vi "cg_Bracket Fletcher.vi"(4 "p":dbl[](array[numeric]) format="%.2f", 6 "loops":u32, 7 "function and data":T1, 8 "error in (no error)":errorcluster, 9 "xit":dbl[](array[numeric]) format="%.2f", 10 "b (start)":dbl format="%.2f", 11 "a (start)":dbl format="%.2f") -> (0 "error out":errorcluster, 1 "c (bracket)":dbl format="%.2f", 2 "b (bracket)":dbl format="%.2f", 3 "a (bracket)":dbl format="%.2f", 5 "number of function calls":i32)   [LabVIEW 2017, in "NI_Gmath.lvlib"]
uses:
  NI_Gmath.lvlib
  ucno_user function ref and data.ctl
  ucno_user objective function ref.ctl
panel:
  out "error":i32
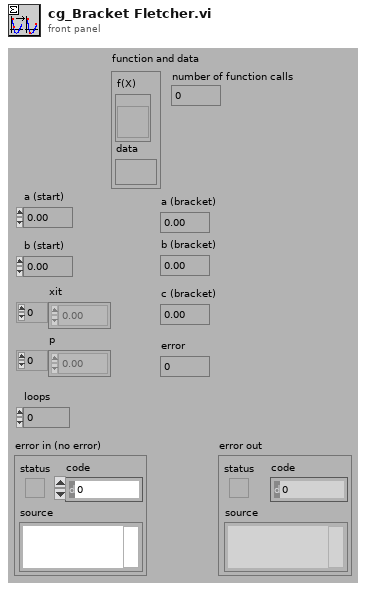
[diagram p1: front panel]
types:
  T1 = typedef "NI_Gmath.lvlib/ucno_user function ref and data.ctl" = cluster{"f(X)":T2, "data":variant}
  T2 = typedef "NI_Gmath.lvlib/ucno_user objective function ref.ctl" = refnum<vi>
  T3 = cluster{"objective function":bool, "gradient":bool}
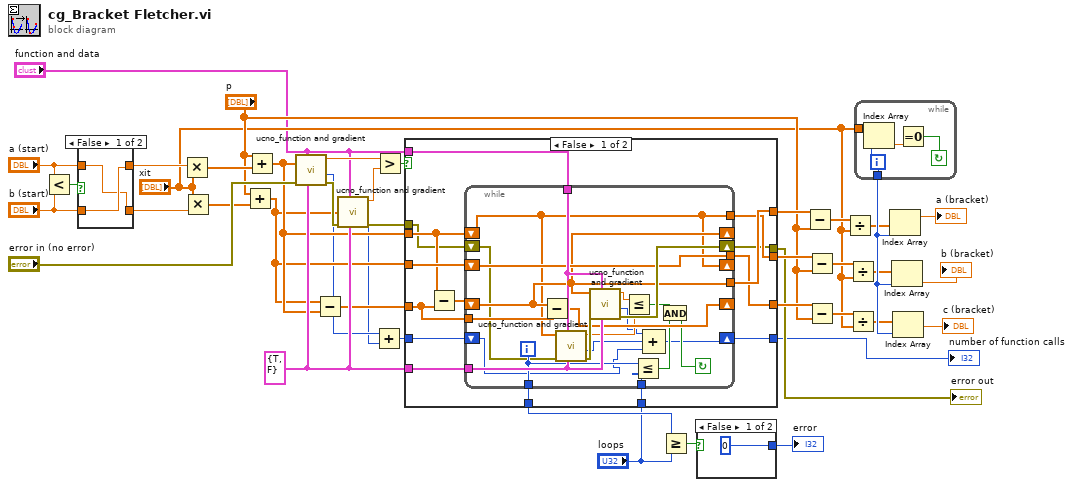
[diagram p0: block diagram]
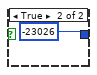
[diagram p3: hidden frame]
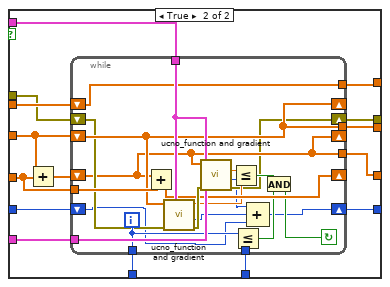
[diagram p4: hidden frame]
diagram:
  w42 = T3 {"objective function"=TRUE, "gradient"=FALSE} ("output control")
  n1 = Less?(x="a (start)", y="b (start)") -> (x < y?=w33:bool)
  n2 = case shown="False" w33 {
    tunnel: "a (start)" -> [w43 w46]
    tunnel: [w44 w46] -> w29
    tunnel: "b (start)" -> [w44 w45]
    tunnel: [w43 w45] -> w26
    frame False {
    }
    frame True {
    }
  }
  n3 = Multiply(x=w29, y="xit") -> (x*y=w28:dbl[])
  n4 = Multiply(x="xit", y=w26) -> (x*y=w25:dbl[])
  n5 = Add(x="p", y=w25) -> (x+y=w24:dbl[])
  n6 = Add(x="p", y=w28) -> (x+y=w27:dbl[])
  n7 = call "ucno_function and gradient.vi"("output control"=w42, "function and data"="function and data", "error in (no error)"="error in (no error)", "X"=w27) -> ("error out"=w41:errorcluster, "number of function calls"=w4:i32, "f(X)"=w8:dbl)  [unwired: 4 in, 1 out]
  n8 = Subtract(x=w24, y=w27) -> (x-y=w38:dbl[])
  n9 = call "ucno_function and gradient.vi"("output control"=w42, "function and data"="function and data", "error in (no error)"=w41, "X"=w24) -> ("error out"=w7:errorcluster, "number of function calls"=w3:i32, "f(X)"=w31:dbl)  [unwired: 4 in, 1 out]
  n10 = Add(x=w4, y=w3) -> (x+y=w2:i32)
  n11 = Greater?(x=w8, y=w31) -> (0:w39:bool)
  n12 = case shown="False" w39 {
    tunnel: w27 -> [w58 w97]
    tunnel: w24 -> [w59 w96]
    tunnel: w38 -> [w56 w94]
    tunnel: [w55 w91] -> w23
    tunnel: [w54 w90] -> w21
    tunnel: [w53 w89] -> w20
    tunnel: [w61 w93] -> w37
    tunnel: "loops" -> [w60 w92]
    tunnel: w7 -> [w52 w88]
    tunnel: [w51 w87] -> w6
    tunnel: "function and data" -> [w50 w86]
    tunnel: w42 -> [w49 w85]
    tunnel: w2 -> [w48 w84]
    tunnel: [w47 w83] -> w1
    frame False {
      n13 = Subtract(x=w58, y=w56) -> (x-y=w57:dbl[])
      n14 = while {
        tunnel: [w71] -> w53
        tunnel: [w69] -> w54
        tunnel: [w70] -> w55
        tunnel: w60 -> [w66]
        tunnel: [w75] -> w61
        tunnel: w56 -> [w78]
        shift-left: w57 -> [w70]
        shift-right: [w76] -> _
        shift-left: w59 -> [w71]
        shift-right: [w69] -> _
        shift-left: w58 -> [w69]
        shift-right: [w70] -> _
        shift-right: [w81] -> w51
        shift-left: w52 -> [w67]
        tunnel: w50 -> [w82]
        tunnel: w49 -> [w80]
        shift-right: [w62] -> w47
        shift-left: w48 -> [w63]
        i -> [w75]
        stop <- w72 continue-if-true
        n15 = Subtract(x=w70, y=w78) -> (x-y=w76:dbl[])
        n16 = call "ucno_function and gradient.vi"("output control"=w80, "function and data"=w82, "error in (no error)"=w67, "X"=w69) -> ("error out"=w79:errorcluster, "number of function calls"=w64:i32, "f(X)"=w68:dbl)  [unwired: 4 in, 1 out]
        n17 = call "ucno_function and gradient.vi"("output control"=w80, "function and data"=w82, "error in (no error)"=w79, "X"=w70) -> ("error out"=w81:errorcluster, "number of function calls"=w65:i32, "f(X)"=w77:dbl)  [unwired: 4 in, 1 out]
        n18 = Less Or Equal?(x=w77, y=w68) -> (x <= y?=w74:bool)
        n19 = Less Or Equal?(x=w75, y=w66) -> (x <= y?=w73:bool)
        n20 = Compound Arithmetic op=ADD(w65, w64, w63) -> (w62:i32)
        n21 = And(x=w74, y=w73) -> (x .and. y?=w72:bool)
      }
    }
    frame True {
      n22 = Add(x=w96, y=w94) -> (x+y=w95:dbl[])
      n23 = while {
        tunnel: [w103] -> w89
        tunnel: [w107] -> w90
        tunnel: [w108] -> w91
        tunnel: w92 -> [w112]
        tunnel: [w113] -> w93
        tunnel: w94 -> [w115]
        shift-left: w95 -> [w103]
        shift-right: [w114] -> _
        shift-left: w96 -> [w107]
        shift-right: [w103] -> _
        shift-left: w97 -> [w108]
        shift-right: [w107] -> _
        shift-right: [w102] -> w87
        shift-left: w88 -> [w105]
        tunnel: w86 -> [w118]
        tunnel: w85 -> [w117]
        shift-right: [w98] -> w83
        shift-left: w84 -> [w99]
        i -> [w113]
        stop <- w109 continue-if-true
        n24 = Add(x=w103, y=w115) -> (x+y=w114:dbl[])
        n25 = call "ucno_function and gradient.vi"("function and data"=w118, "error in (no error)"=w105, "X"=w107) -> ("error out"=w116:errorcluster, "number of function calls"=w100:i32, "f(X)"=w106:dbl)  [unwired: 5 in, 1 out]
        n26 = call "ucno_function and gradient.vi"("output control"=w117, "function and data"=w118, "error in (no error)"=w116, "X"=w103) -> ("error out"=w102:errorcluster, "number of function calls"=w101:i32, "f(X)"=w104:dbl)  [unwired: 4 in, 1 out]
        n27 = Less Or Equal?(x=w104, y=w106) -> (x <= y?=w111:bool)
        n28 = Less Or Equal?(x=w113, y=w112) -> (x <= y?=w110:bool)
        n29 = Compound Arithmetic op=ADD(w101, w100, w99) -> (w98:i32)
        n30 = And(x=w111, y=w110) -> (x .and. y?=w109:bool)
      }
    }
  }
  "error out" <- w6
  "number of function calls" <- w1
  n31 = Greater Or Equal?(x=w37, y="loops") -> (x >= y?=w35:bool)
  n32 = case shown="False" w35 {
    tunnel: [0 -23026] -> w34
    frame False {
    }
    frame True {
    }
  }
  "error" <- w34
  n33 = Subtract(x=w23, y="p") -> (x-y=w22:dbl[])
  n34 = Subtract(x=w21, y="p") -> (x-y=w18:dbl[])
  n35 = Subtract(x=w20, y="p") -> (x-y=w17:dbl[])
  n36 = Divide(x=w22, y="xit") -> (x/y=w14:dbl[])
  n37 = Divide(x=w18, y="xit") -> (x/y=w13:dbl[])
  n38 = Divide(x=w17, y="xit") -> (x/y=w12:dbl[])
  n39 = while {
    tunnel: [w123] -> w15
    tunnel: "xit" -> [w124]
    i -> [w123]
    stop <- w121 continue-if-true
    n40 = Index Array(array=w124, index=w123) -> (element=w122:dbl)
    n41 = Equal To 0?(x=w122) -> (x = 0?=w121:bool)
  }
  n42 = Index Array(array=w14, index=w15) -> (element=→"a (bracket)":dbl)
  n43 = Index Array(array=w13, index=w15) -> (element=→"b (bracket)":dbl)
  n44 = Index Array(array=w12, index=w15) -> (element=→"c (bracket)":dbl)
